vi "Verlustmoment.vi"(8 "n [1/min":dbl, 9 "Verlustmoment M0 [Nm] bei n = 0":dbl, 10 "Verlustmoment M1 [Nm] bei n1":dbl, 11 "Rollendrehzahl n1 [1/min]":u16=1 min=1) -> (3 "Mv":dbl)   [LabVIEW 2014]
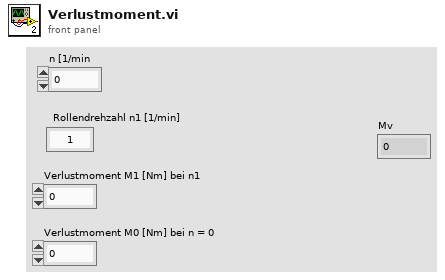
[diagram p1: front panel]
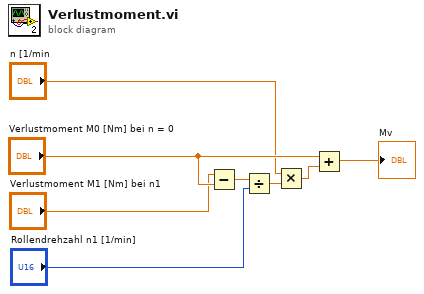
[diagram p0: block diagram]
diagram:
  n1 = Subtract(x="Verlustmoment M1 [Nm] bei n1", y="Verlustmoment M0 [Nm] bei n = 0") -> (x-y=w6:dbl)
  n2 = Divide(x=w6, y="Rollendrehzahl n1 [1/min]") -> (x/y=w7:dbl)
  n3 = Multiply(x="n [1/min", y=w7) -> (x*y=w8:dbl)
  n4 = Add(x="Verlustmoment M0 [Nm] bei n = 0", y=w8) -> (x+y=→"Mv":dbl)
